vi "Open Picture.vi"(8 "Error In":errorcluster, 11 "Picture Path":path) -> (0 "Error Out":errorcluster, 2 "Image":T1)   [LabVIEW 2016]
doc: "Creates image cluster from image at given path\n\nError 5000: Image Not PNG or JPEG\nError 5001: Not 8-Bit Image"
uses:
  <vilib>/picture/picture.llb/imagedata.ctl
  <vilib>/Utility/error.llb/Error Cluster From Error Code.vi
  <vilib>/ErrorRing/Error Ring.xnode
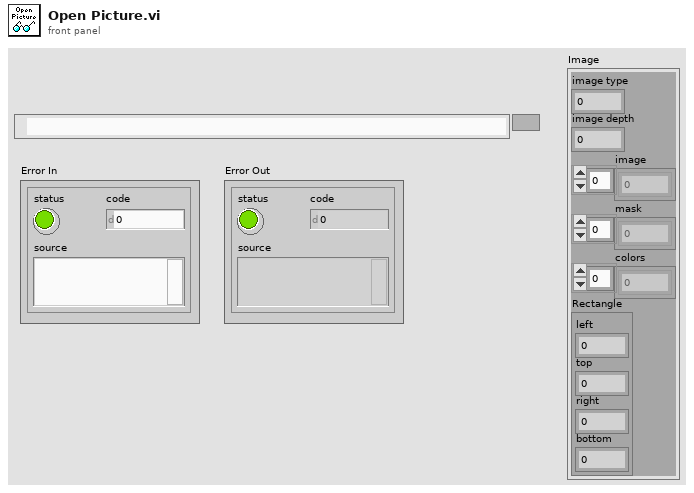
[diagram p1: front panel]
types:
  T1 = typedef "imagedata.ctl" = cluster{"image type":i32, "image depth":i32, "image":u8[], "mask":u8[], "colors":u32[], "Rectangle":cluster{"left":i16, "top":i16, "right":i16, "bottom":i16}}
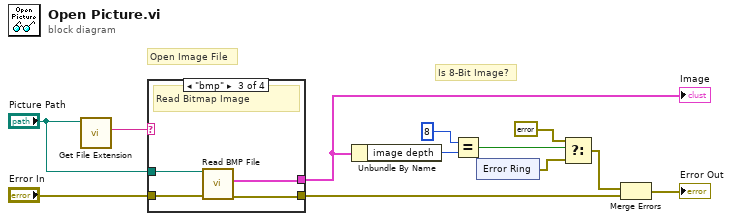
[diagram p0: block diagram]
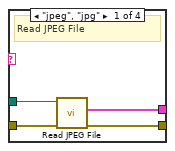
[diagram p2: hidden frame]
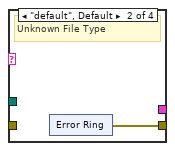
[diagram p3: hidden frame]
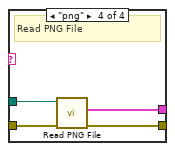
[diagram p4: hidden frame]
diagram:
  # "Is 8-Bit Image?"
  # "Open Image File"
  n1 = call <vilib>:"Get File Extension.vi"("file"="Picture Path") -> ("lowercase file extension"=w2:string)  [unwired: 6 in, 4 out]
  n2 = case shown="\"bmp\"" w2 {
    tunnel: "Picture Path" -> [w16 _ w26 w30]
    tunnel: "Error In" -> [w15 _ w25 w29]
    tunnel: [w14 w17 w23 w27] -> w3
    tunnel: [w13 _ w24 w28] -> w11
    frame "jpeg", "jpg" {
      # "Read JPEG File"
      n3 = call <vilib>:"Read JPEG File.vi"("error in (no error)"=w15, "path to JPEG file"=w16) -> ("error out"=w14:errorcluster, "image data"=w13:T1)  [unwired: 7 in, 1 out]
    }
    frame "default", Default {
      # "Unknown File Type"
      n4 = xnode "Error Ring"() -> ("error out"=w17:errorcluster)
    }
    frame "bmp" {
      # "Read Bitmap Image"
      n5 = call <vilib>:"Read BMP File.vi"("error in (no error)"=w25, "path to BMP file"=w26) -> ("error out"=w23:errorcluster, "image data"=w24:T1)  [unwired: 7 in, 1 out]
    }
    frame "png" {
      # "Read PNG File"
      n6 = call <vilib>:"Read PNG File.vi"("error in (no error)"=w29, "path to PNG file"=w30) -> ("error out"=w27:errorcluster, "image data"=w28:T1)  [unwired: 7 in, 1 out]
    }
  }
  "Image" <- w11
  n7 = Unbundle By Name(w11) -> ("image depth"=w10:i32)
  n8 = Equal?(x=8, y=w10) -> (x = y?=w6:bool)
  n9 = xnode "Error Ring"() -> ("error out"=w7:errorcluster)
  n10 = Select(t=errorcluster {"status"=FALSE, "code"=0, "source"=""} ("error constant"), s=w6, f=w7) -> (s? t:f=w4:errorcluster)
  n11 = Merge Errors(w4, w3) -> (→"Error Out":errorcluster)
